vi "Plant Simulator.vi"(0 "Initial PV":dbl format="%.2f", 1 "dt (s)":dbl=-1.0 format="%.3f", 2 "Measurement Noise (%)":dbl(slide) scale=0.0..100.0, 4 "Controller Noise (%)":dbl(slide) scale=0.0..100.0, 5 "Valve Deadband":dbl format="%.1f", 6 "Process Deadtime":i32(slide) scale=0.0..5.0, 7 "Lag (min)":dbl format="%.2f", 8 "Process Load":dbl(slide) scale=0.0..50.0, 9 "Process Gain":dbl(slide)=1.0 scale=0.0..5.0, 10 "Manipulated Variable (Output, %)":dbl format="%.2f", 11 "iteration":i32) -> (3 "Process Variable (%)":dbl format="%.2f")   [LabVIEW 2010]
doc: "Simulates a physical plant's response; for use with feedback control loops.\n\nAll scale factors are in percent. Lag time is in minutes. Process Deadtime is a true deadtime, measured as a multiple of the loop cycle time. NOTE: this deadtime is dependent upon the interval at which this VI is called. You can modify the algorithm used here to simulate almost any process.\n\nIf more than one plant needs to be simulated simultaneously, save multiple copies of this VI under different names."
panel:
  # "Plant Characteristics"
  # "(x cycle time)"
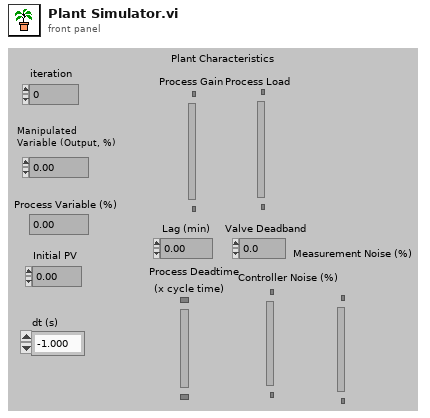
[diagram p1: front panel]
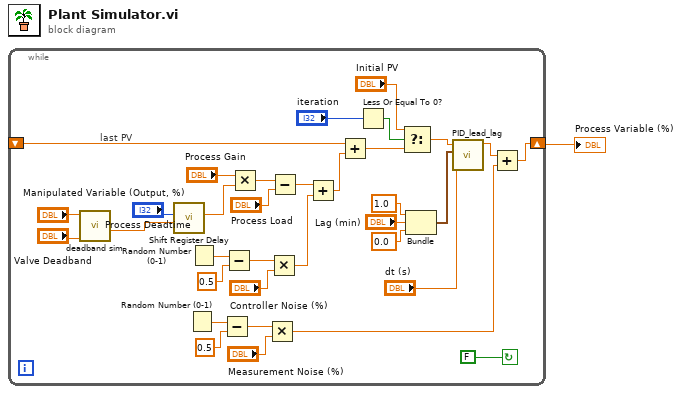
[diagram p0: block diagram]
diagram:
  n1 = while {
    shift-left: _ -> [w12]
    shift-right: [w7] -> w1
    stop <- FALSE continue-if-true
    # "last PV"
    n2 = call "deadband sim.vi"("Deadband (%)"="Valve Deadband", "requested pos. (%)"="Manipulated Variable (Output, %)") -> ("actual pos. (%)"=w35:dbl)  [unwired: 9 in]
    n3 = call "Shift Register Delay.vi"("input"=w35, "n delay(0)"="Process Deadtime") -> ("output"=w31:dbl)  [unwired: 9 in]
    n4 = Random Number (0-1)() -> (number: 0 to 1=w11:dbl)
    n5 = Random Number (0-1)() -> (number: 0 to 1=w21:dbl)
    n6 = Subtract(x=w11, y=0.5) -> (x-y=w9:dbl)
    n7 = Subtract(x=w21, y=0.5) -> (x-y=w28:dbl)
    n8 = Multiply(x="Process Gain", y=w31) -> (x*y=w22:dbl)
    n9 = Multiply(x=w9, y="Measurement Noise (%)") -> (x*y=w6:dbl)
    n10 = Multiply(x=w28, y="Controller Noise (%)") -> (x*y=w34:dbl)
    n11 = Subtract(x=w22, y="Process Load") -> (x-y=w23:dbl)
    n12 = Add(x=w23, y=w34) -> (x+y=w27:dbl)
    n13 = Add(x=w12, y=w27) -> (x+y=w17:dbl)
    n14 = Less Or Equal To 0?(x="iteration") -> (x <= 0?=w16:bool)
    n15 = Select(t="Initial PV", s=w16, f=w17) -> (s? t:f=w5:dbl)
    n16 = Bundle(1.0, "Lag (min)"="Lag (min)", 0.0) -> (w3:cluster{dbl, "Lag (min)":dbl, dbl})  [unwired: 1 in]
    n17 = call "PID_lead_lag.vi"("dt (s) in"="dt (s)", "Tuning parameters"=w3, "Input"=w5) -> ("Output"=w4:dbl)  [unwired: 8 in]
    n18 = Add(x=w4, y=w6) -> (x+y=w7:dbl)
  }
  "Process Variable (%)" <- w1
